vi "_emi_GFV System colors.vi"(1 "Action(GET)":enum16{"GET", "SET"}(ring), 7 "System background in":T1={"Main Top Panels"={"Type"=enum."FlatColor", "Dark/Primary Color"=0, "Light/Secondary Color"=11776947, "Extra Color"=0}, "Main Botom Panels"={"Type"=enum."FlatColor", "Dark/Primary Color"=0, "Light/Secondary Color"=11776947, "Extra Color"=0}, "Graphs"={"Type"=enum."FlatColor", "Dark/Primary Color"=0, "Light/Secondary Color"=11776947, "Extra Color"=0}, "Dialogs"={"Type"=enum."FlatColor", "Dark/Primary Color"=0, "Light/Secondary Color"=11776947, "Extra Color"=0}}, 11 "error in (no error)":errorcluster) -> (8 "System background out":T1={"Main Top Panels"={"Type"=enum."FlatColor", "Dark/Primary Color"=0, "Light/Secondary Color"=11776947, "Extra Color"=0}, "Main Botom Panels"={"Type"=enum."FlatColor", "Dark/Primary Color"=0, "Light/Secondary Color"=11776947, "Extra Color"=0}, "Graphs"={"Type"=enum."FlatColor", "Dark/Primary Color"=0, "Light/Secondary Color"=11776947, "Extra Color"=0}, "Dialogs"={"Type"=enum."FlatColor", "Dark/Primary Color"=0, "Light/Secondary Color"=11776947, "Extra Color"=0}}, 15 "error out":errorcluster)   [LabVIEW 2011]
uses:
  emi_System Colors.ctl
  _emi_ Color defenition.ctl
  Basic/0 - General/Graphix/Private/emi_List Of Graphix.ctl
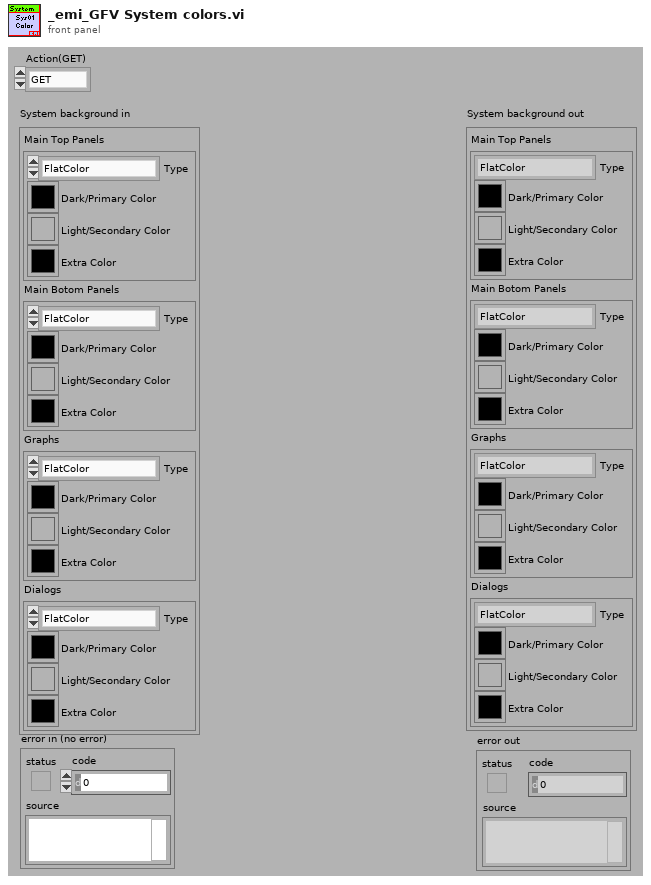
[diagram p1: front panel]
types:
  T1 = typedef "emi_System Colors.ctl" = cluster{"Main Top Panels":T2, "Main Botom Panels":T2, "Graphs":T2, "Dialogs":T2}
  T2 = typedef "_emi_ Color defenition.ctl" = cluster{"Type":T3, "Dark/Primary Color":u32, "Light/Secondary Color":u32, "Extra Color":u32}
  T3 = typedef "emi_List Of Graphix.ctl" = enum16{"FlatColor", "SharpGrad", "ShallowGrad", "GlasGradBord", "GlasGrad", "GlasGradBord 2"}
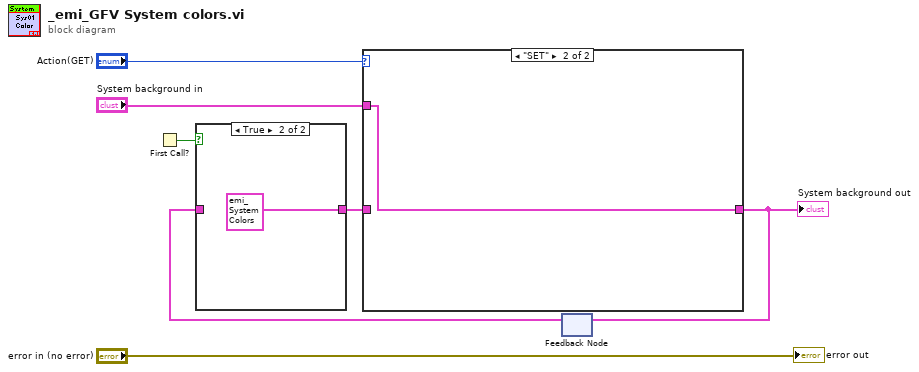
[diagram p0: block diagram]
diagram:
  n1 = First Call?() -> (First Call?: T/F=w4:bool)
  n2 = feedback #1() -> (w5:T1)  [unwired: 1 in]
  n3 = case shown="True" w4 {
    tunnel: w5 -> [w8 _]
    tunnel: [w8 T1 {"Main Top Panels"={"Type"=enum."GlasGradBord 2", "Dark/Primary Color"=0, "Light/Secondary Color"=11776947, "Extra Color"=0}, "Main Botom Panels"={"Type"=enum."FlatColor", "Dark/Primary Color"=11776947, "Light/Secondary Color"=11776947, "Extra Color"=0}, "Graphs"={"Type"=enum."FlatColor", "Dark/Primary Color"=0, "Light/Secondary Color"=0, "Extra Color"=11776947}, "Dialogs"={"Type"=enum."FlatColor", "Dark/Primary Color"=16448250, "Light/Secondary Color"=16448250, "Extra Color"=0}} ("System background")] -> w2
    frame False {
    }
    frame True {
    }
  }
  n4 = case shown="\"SET\"" "Action(GET)" {
    tunnel: [w10 w11] -> w3
    tunnel: w2 -> [w10 _]
    tunnel: "System background in" -> [_ w11]
    frame "GET", Default {
    }
    frame "SET" {
    }
  }
  "System background out" <- w3
  n5 = feedback-in #1(w3) -> ()
  "error out" <- "error in (no error)"
